vi "Break_Loop_State_Control.vi"(8 "Error In":errorcluster, 9 "Control Reference Cluster Input":T1, 11 "Control State In":T2(ring)=enum."Disabled and Grayed Out") -> (0 "error out":errorcluster, 3 "Break Loop RefNum":refnum<vi>)   [LabVIEW 2016]
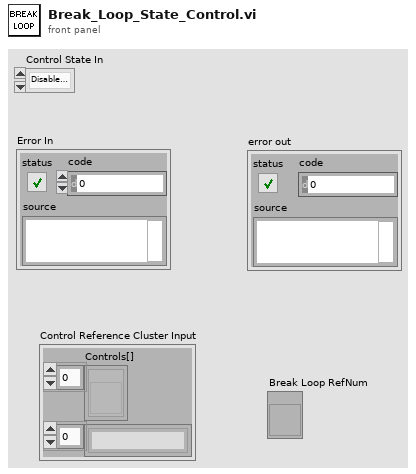
[diagram p1: front panel]
types:
  T1 = cluster{"Controls[]":refnum<vi>[], "Control Names":string[]}
  T2 = enum8{"Enabled", "Disabled", "Disabled and Grayed Out"}
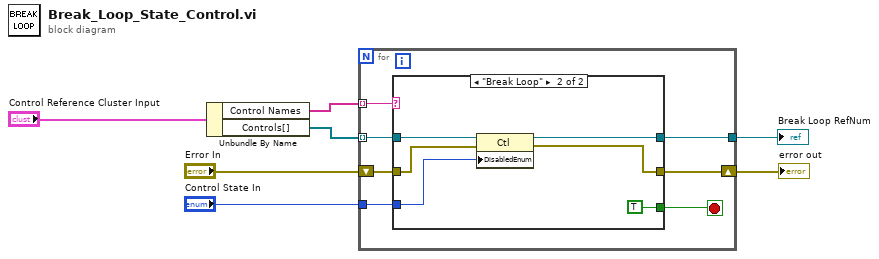
[diagram p0: block diagram]
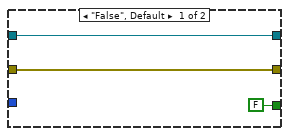
[diagram p2: hidden frame]
diagram:
  n1 = Unbundle By Name("Control Reference Cluster Input") -> ("Control Names"=w4:string[], "Controls[]"=w3:refnum<vi>[])
  n2 = for {
    tunnel: w4 -> [w14] mode=indexing
    tunnel: "Control State In" -> [w12]
    shift-right: [w9] -> w5
    shift-left: "Error In" -> [w10]
    tunnel: w3 -> [w13] mode=indexing
    tunnel: [w11] -> w1
    stop <- w8 stop-if-true
    n3 = case shown="\"Break Loop\"" w14 {
      tunnel: w13 -> [w17 w20]
      tunnel: w12 -> [_ w23]
      tunnel: [w17 w19] -> w11
      tunnel: w10 -> [w16 w22]
      tunnel: [w16 w21] -> w9
      tunnel: [FALSE TRUE] -> w8
      frame "False", Default {
      }
      frame "Break Loop" {
        n4 = property class="Ctl"(reference=w20, error in=w22, "DisabledEnum"=w23) -> (reference out=w19:refnum<vi>, error out=w21:errorcluster)
      }
    }
  }
  "error out" <- w5
  "Break Loop RefNum" <- w1
